vi "Config_SaveKeys.vi"(8 "error in (no error)":errorcluster, 9 "Configuration Save":T1={"General"={"Config.ini"=path "", "Default Logging Path"=path ""}, "Hardware"={"Global T VAR"="", "Global B VAR"="", "VISAS"={"GEN COM"="", "SCOPE COM"="", "VNA COM"=""}, "Connected?"={"SCOPE"=FALSE, "GEN"=FALSE, "VNA"=FALSE}}, "Operation"={"Operation Mode"=enum."Idle-Off", "Status"="", "NewLog?"=FALSE, "OvenWarn"=FALSE, "Scope Settings"={"TimeBase"=0.0, "VerticalScale"=4.0, "Channel"=enum."Channel 2"}, "Gen Settings"={"Amplitude"=0.0, "Frequency"=0.0, "Offset"=0.0}}}, 10 "Configuration Cluster":T1={"General"={"Config.ini"=path "", "Default Logging Path"=path ""}, "Hardware"={"Global T VAR"="", "Global B VAR"="", "VISAS"={"GEN COM"="", "SCOPE COM"="", "VNA COM"=""}, "Connected?"={"SCOPE"=FALSE, "GEN"=FALSE, "VNA"=FALSE}}, "Operation"={"Operation Mode"=enum."Idle-Off", "Status"="", "NewLog?"=FALSE, "OvenWarn"=FALSE, "Scope Settings"={"TimeBase"=0.0, "VerticalScale"=4.0, "Channel"=enum."Channel 2"}, "Gen Settings"={"Amplitude"=0.0, "Frequency"=0.0, "Offset"=0.0}}}, 11 "Config In":T3) -> (0 "error out":errorcluster, 2 "output cluster":T1={"General"={"Config.ini"=path "", "Default Logging Path"=path ""}, "Hardware"={"Global T VAR"="", "Global B VAR"="", "VISAS"={"GEN COM"="", "SCOPE COM"="", "VNA COM"=""}, "Connected?"={"SCOPE"=FALSE, "GEN"=FALSE, "VNA"=FALSE}}, "Operation"={"Operation Mode"=enum."Idle-Off", "Status"="", "NewLog?"=FALSE, "OvenWarn"=FALSE, "Scope Settings"={"TimeBase"=0.0, "VerticalScale"=4.0, "Channel"=enum."Channel 2"}, "Gen Settings"={"Amplitude"=0.0, "Frequency"=0.0, "Offset"=0.0}}}, 3 "refnum out":T3)   [LabVIEW 2021]
uses:
  <vilib>/Utility/config.llb/Config Data RefNum.ctl
  Config_Cluster.ctl
  Mode_Enum.ctl
  <vilib>/Utility/config.llb/Write Key (Path).vi
  <vilib>/Utility/config.llb/Write Key (String).vi
  <vilib>/Utility/config.llb/NI_LVConfig.lvlib
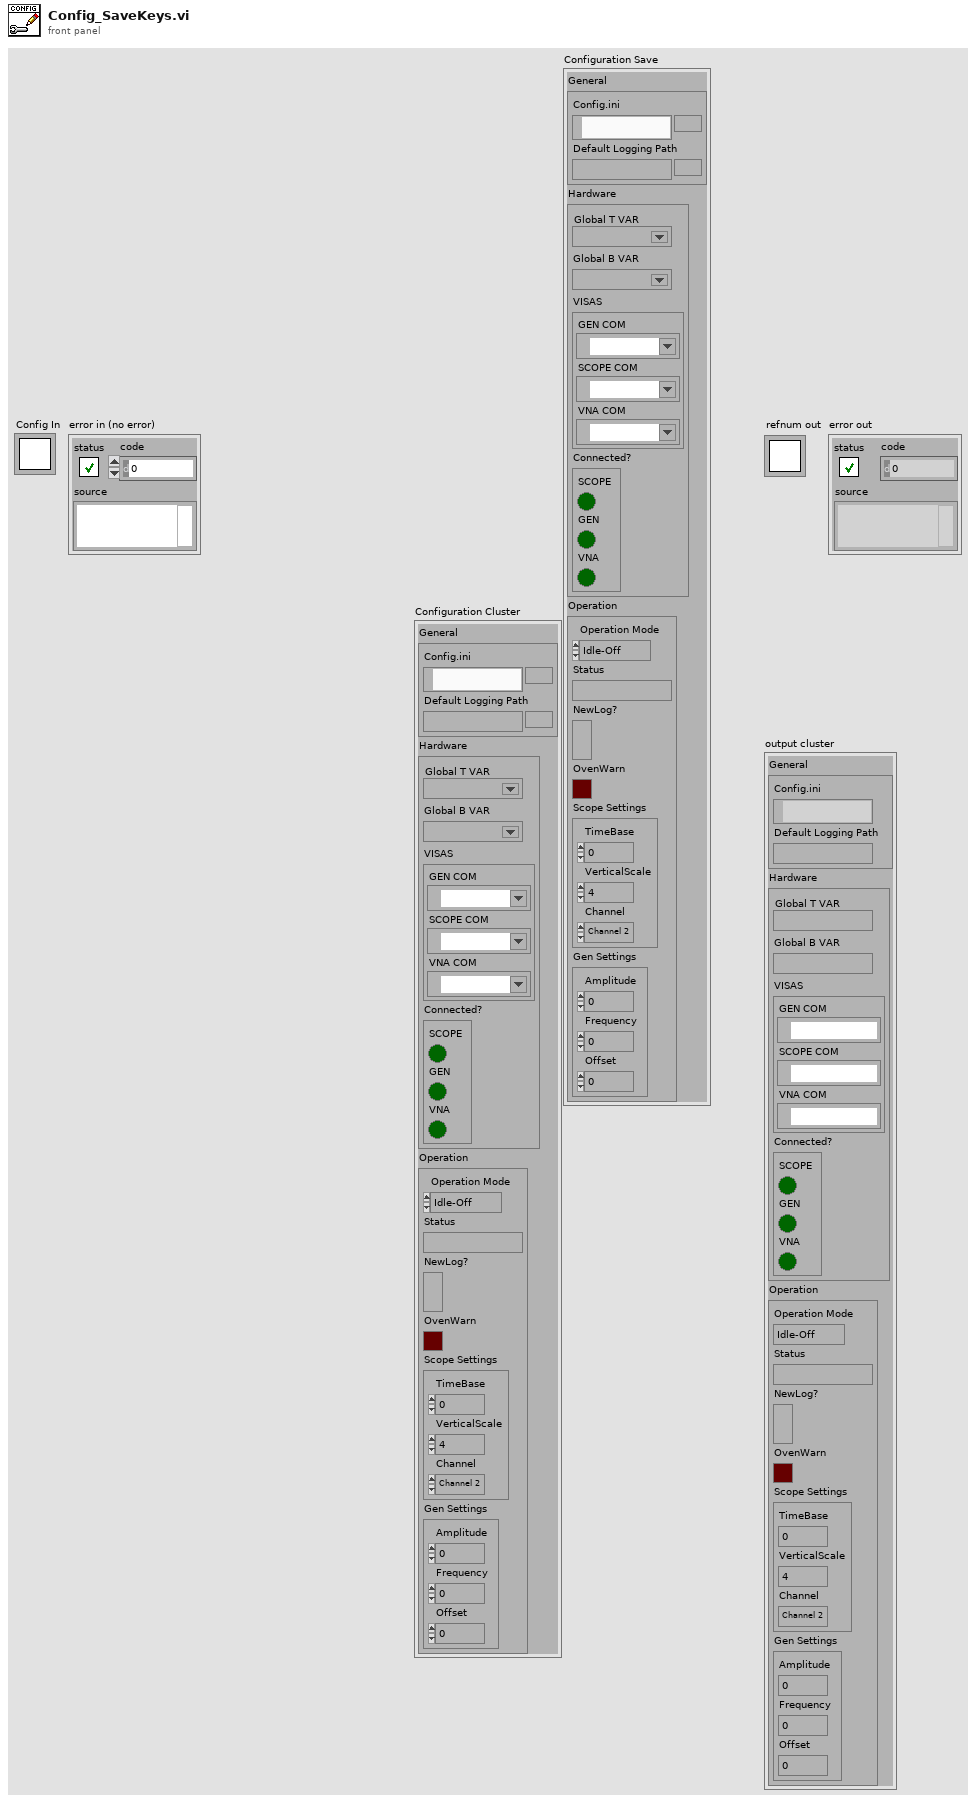
[diagram p1: front panel]
types:
  T1 = typedef "Config_Cluster.ctl" = cluster{"General":cluster{"Config.ini":path, "Default Logging Path":path}, "Hardware":cluster{"Global T VAR":refnum<k21>, "Global B VAR":refnum<k21>, "VISAS":cluster{"GEN COM":refnum<visa-resource-name>, "SCOPE COM":refnum<visa-resource-name>, "VNA COM":refnum<visa-resource-name>}, "Connected?":cluster{"SCOPE":bool, "GEN":bool, "VNA":bool}}, "Operation":cluster{"Operation Mode":T2, "Status":string, "NewLog?":bool, "OvenWarn":bool, "Scope Settings":cluster{"TimeBase":dbl, "VerticalScale":dbl, "Channel":enum16{"Channel 2", "Channel 1"}}, "Gen Settings":cluster{"Amplitude":dbl, "Frequency":dbl, "Offset":dbl}}}
  T2 = typedef "Mode_Enum.ctl" = enum16{"Logging", "Idle-Off", "Idle"}
  T3 = typedef "NI_LVConfig.lvlib/Config Data RefNum.ctl" = refnum<k1>
  T4 = cluster{"GEN COM":refnum<visa-resource-name>, "SCOPE COM":refnum<visa-resource-name>, "VNA COM":refnum<visa-resource-name>}
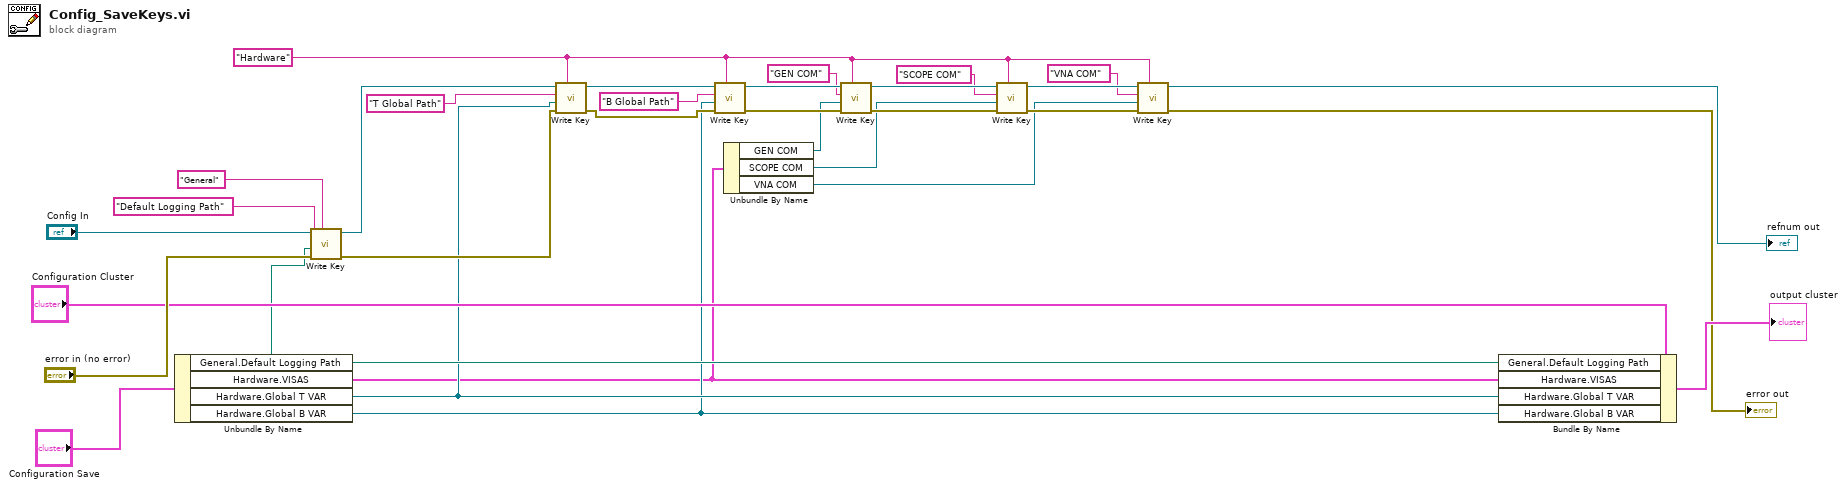
[diagram p0: block diagram]
diagram:
  w10 = "Hardware" ("section")
  n1 = Unbundle By Name("Configuration Save") -> ("General.Default Logging Path"=w19:path, "Hardware.VISAS"=w3:T4, "Hardware.Global T VAR"=w18:refnum<k21>, "Hardware.Global B VAR"=w17:refnum<k21>)
  n2 = call-poly <vilib>:"Write Key.vi"("section"="General", "error in (no error)"="error in (no error)", "value"=w19, "key"="Default Logging Path", "refnum"="Config In") -> ("error out"=w21:errorcluster, "refnum out"=w22:T3)  [unwired: 4 in, 1 out]
  n3 = call-poly <vilib>:"Write Key.vi"("section"=w10, "error in (no error)"=w21, "value"=w18, "key"="T Global Path", "refnum"=w22) -> ("error out"=w23:errorcluster, "refnum out"=w26:T3)  [unwired: 4 in, 1 out]
  n4 = call-poly <vilib>:"Write Key.vi"("section"=w10, "error in (no error)"=w23, "value"=w17, "key"="B Global Path", "refnum"=w26) -> ("error out"=w7:errorcluster, "refnum out"=w16:T3)  [unwired: 4 in, 1 out]
  n5 = Unbundle By Name(w3) -> ("GEN COM"=w6:refnum<visa-resource-name>, "SCOPE COM"=w5:refnum<visa-resource-name>, "VNA COM"=w4:refnum<visa-resource-name>)
  n6 = call-poly <vilib>:"Write Key.vi"("section"=w10, "error in (no error)"=w7, "value"=w6, "key"="GEN COM", "refnum"=w16) -> ("error out"=w8:errorcluster, "refnum out"=w15:T3)  [unwired: 4 in, 1 out]
  n7 = call-poly <vilib>:"Write Key.vi"("section"=w10, "error in (no error)"=w8, "value"=w5, "key"="SCOPE COM", "refnum"=w15) -> ("error out"=w9:errorcluster, "refnum out"=w14:T3)  [unwired: 4 in, 1 out]
  n8 = call-poly <vilib>:"Write Key.vi"("section"=w10, "error in (no error)"=w9, "value"=w4, "key"="VNA COM", "refnum"=w14) -> ("error out"=→"error out":errorcluster, "refnum out"=→"refnum out":T3)  [unwired: 4 in, 1 out]
  n9 = Bundle By Name(cluster="Configuration Cluster", "General.Default Logging Path"=w19, "Hardware.VISAS"=w3, "Hardware.Global T VAR"=w18, "Hardware.Global B VAR"=w17) -> (→"output cluster":T1)
